vi "NI VeriStand - Open Single Waveform Write Session (DBL).vi"(7 "Communication Properties":T2, 8 "error in (no error)":errorcluster, 10 "dt":dbl=nan, 11 "DBL Waveform Data Reference":T1) -> (0 "error out":errorcluster, 3 "Single Waveform Write Session (DBL)":refnum<class "Single Waveform Write (DBL).lvclass">)   [LabVIEW 2020, in "NI_VS Custom Device Waveform API.lvlib" / "Single Waveform Write (DBL).lvclass"]
doc: "Opens a session for reading data from or writing data to a specific waveform or waveforms associated with a custom device. You must manually select the instance to use according to the number of waveforms with which you want to interact, whether the data type of the waveforms is DBL or CDB, and whether you want to read or write waveform data."
uses:
  Single Waveform Write (DBL).lvclass
  D:/p4/penguin/lvaddon/Veristand/master/src/LabVIEW/vilib/NI VeriStand/Custom Device Waveform API/Waveform Session.lvclass
  Communication Properties.ctl
  Custom Device API/Waveform Data Reference.ctl
  Access mode.ctl
  Internal Comm Classes/WPL Comm/WPL Comm (1D DBL)/WPL Comm (1D DBL).lvclass
  Single Waveform Write (DBL).lvclass/Single Waveform Write (DBL).ctl
  Waveform Session.lvclass/Waveform Session.ctl
  Waveform Session.lvclass
  NI_VS Custom Device Waveform API.lvlib
  Custom Device API/Custom Device API.lvlib
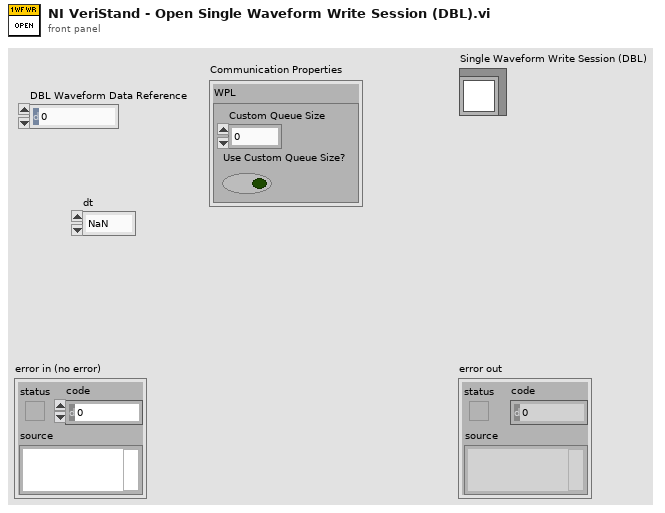
[diagram p1: front panel]
types:
  T1 = typedef "Custom Device API.lvlib/Waveform Data Reference.ctl" = i32
  T2 = typedef "NI_VS Custom Device Waveform API.lvlib/Communication Properties.ctl" = cluster{"WPL":cluster{"Custom Queue Size":i32, "Use Custom Queue Size?":bool}}
  T3 = typedef "NI_VS Custom Device Waveform API.lvlib/Access mode.ctl" = enum16{"Read", "Write"}
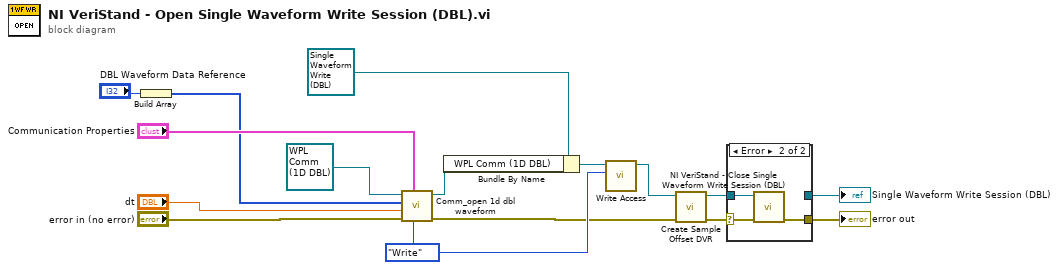
[diagram p0: block diagram]
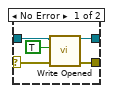
[diagram p2: hidden frame]
diagram:
  w13 = Access_mode."Write" ("Access")
  n1 = Build Array("DBL Waveform Data Reference") -> (w1:T1[])
  n2 = call "Comm_open 1d dbl waveform.vi"("Access"=w13, "Communication Properties"="Communication Properties", "error in (no error)"="error in (no error)", "dt"="dt", "WFM Data Ref"=w1, "WPL Comm (1D DBL) in"=refnum<class "WPL Comm (1D DBL).lvclass"> refnum ("Internal Comm Classes.lvlib:WPL Comm (1D DBL).lvclass")) -> ("error out"=w12:errorcluster, "WPL Comm (1D DBL) out"=w5:refnum<class "WPL Comm (1D DBL).lvclass">)  [unwired: 4 in]
  n3 = Bundle By Name(cluster=refnum<class "Single Waveform Write (DBL).lvclass"> refnum, "WPL Comm (1D DBL)"=w5) -> (w4:refnum<class "Single Waveform Write (DBL).lvclass">)
  n4 = call "Write Access.vi"("Access"=w13, "Waveform Session in"=w4) -> ("Waveform Session out"=w9:refnum<class "Single Waveform Write (DBL).lvclass">)  [unwired: 9 in]
  n5 = call "Create Sample Offset DVR.vi"("error in (no error)"=w12, "Waveform Session in"=w9) -> ("error out"=w10:errorcluster, "Waveform Session out"=w11:refnum<class "Single Waveform Write (DBL).lvclass">)  [unwired: 8 in]
  n6 = case shown="Error" w10 {
    selector: w10 -> [w20 w23]
    tunnel: [w20 w22] -> w16
    tunnel: w11 -> [w19 w21]
    tunnel: [w18 _] -> w14
    frame No Error {
      n7 = call "Write Opened.vi"("Opened"=TRUE, "Waveform Session in"=w19) -> ("Waveform Session out"=w18:refnum<class "Single Waveform Write (DBL).lvclass">)  [unwired: 9 in]
    }
    frame Error {
      n8 = call "NI VeriStand - Close Single Waveform Write Session (DBL).vi"("error in (no error)"=w23, "Single Waveform Write Session (DBL)"=w21) -> ("error out"=w22:errorcluster)  [unwired: 9 in]
    }
  }
  "error out" <- w16
  "Single Waveform Write Session (DBL)" <- w14
